vi "CRYSet Sequence Generator Front Panel.vi"(11 "Vi Ref In":refnum<vi> caption="Vi Ref") -> (3 "Vi Ref Out":refnum<vi> caption="Vi Ref")   [LabVIEW 2013]
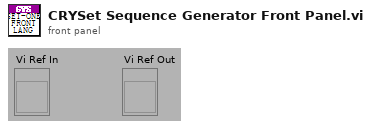
[diagram p1: front panel]
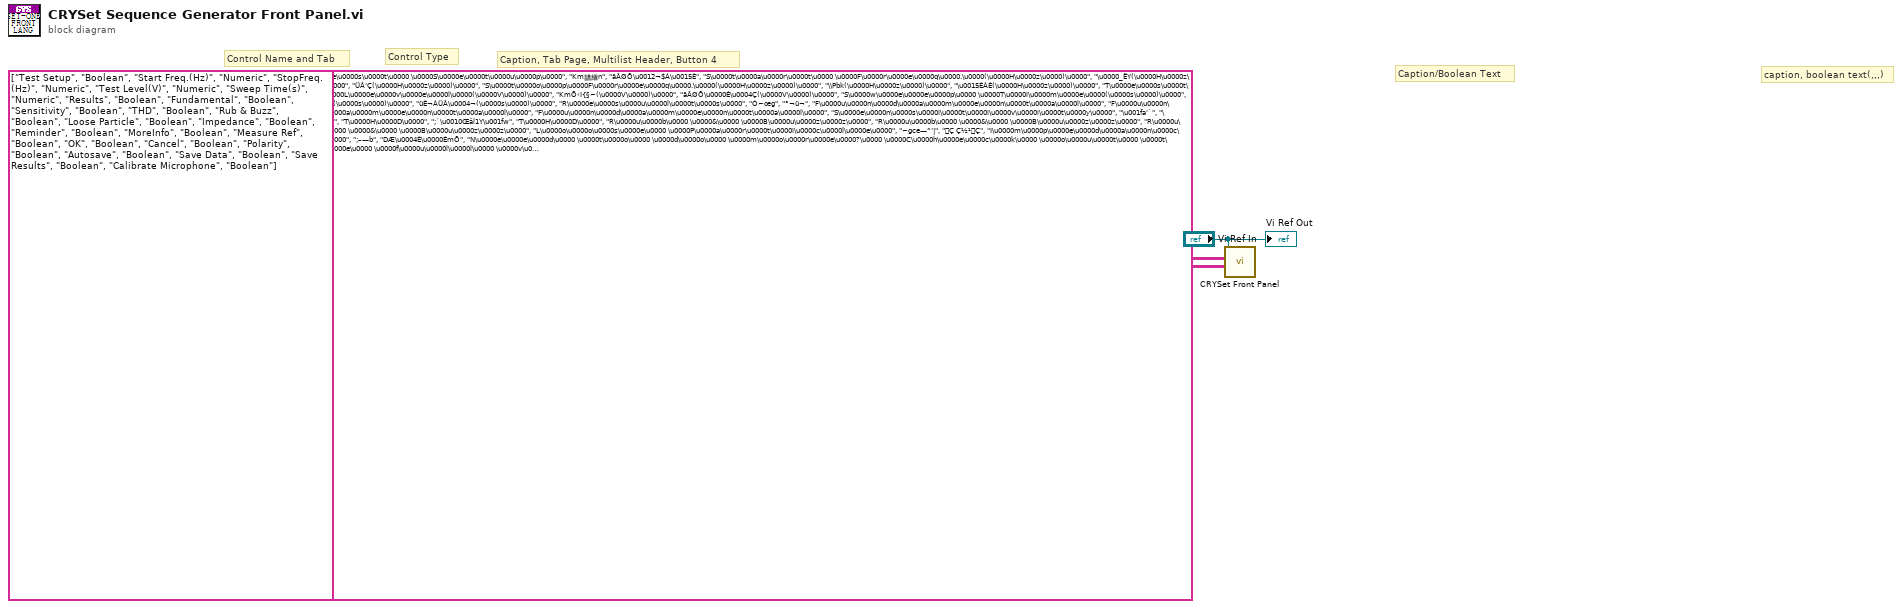
[diagram p0: block diagram]
diagram:
  # "Caption, Tab Page, Multilist Header, Button 4"
  # "Control Type"
  # "Control Name and Tab"
  # "caption, boolean text(,,,)"
  # "Caption/Boolean Text"
  n1 = call "CRYSet Front Panel.vi"("Caption(Boolean Text)"=string[][] [["T\u0000e\u0000s\u0000t\u0000 \u0000S\u0000e\u0000t\u0000u\u0000p\u0000", "Km諎緥n", "äÂØÕ\u0012¬$Á\u0015È"], ["S\u0000t\u0000a\u0000r\u0000t\u0000 \u0000F\u0000r\u0000e\u0000q\u0000.\u0000(\u0000H\u0000z\u0000)\u0000", "\u0000_ËY(\u0000H\u0000z\u0000)\u0000", "ÜÂ‘Ç(\u0000H\u0000z\u0000)\u0000"], ["S\u0000t\u0000o\u0000p\u0000F\u0000r\u0000e\u0000q\u0000.\u0000(\u0000H\u0000z\u0000)\u0000", "\\Pbk(\u0000H\u0000z\u0000)\u0000", "\u0015ÈÀÉ(\u0000H\u0000z\u0000)\u0000"], ["T\u0000e\u0000s\u0000t\u0000 \u0000L\u0000e\u0000v\u0000e\u0000l\u0000(\u0000V\u0000)\u0000", "KmÕ‹I{§~(\u0000V\u0000)\u0000", "äÂØÕ\u0000É\u0004Ç(\u0000V\u0000)\u0000"], ["S\u0000w\u0000e\u0000e\u0000p\u0000 \u0000T\u0000i\u0000m\u0000e\u0000(\u0000s\u0000)\u0000", "kbÏcöeô•(\u0000s\u0000)\u0000", "üÈ¬ÀÜÂ\u0004¬(\u0000s\u0000)\u0000"], ["R\u0000e\u0000s\u0000u\u0000l\u0000t\u0000s\u0000", "Ó~œg", "°¬ü¬"], ["F\u0000u\u0000n\u0000d\u0000a\u0000m\u0000e\u0000n\u0000t\u0000a\u0000l\u0000", "F\u0000u\u0000n\u0000d\u0000a\u0000m\u0000e\u0000n\u0000t\u0000a\u0000l\u0000", "F\u0000u\u0000n\u0000d\u0000a\u0000m\u0000e\u0000n\u0000t\u0000a\u0000l\u0000"], ["S\u0000e\u0000n\u0000s\u0000i\u0000t\u0000i\u0000v\u0000i\u0000t\u0000y\u0000", "\u001fa'`", "\u0010¬Ä³"], ["T\u0000H\u0000D\u0000", ";`\u0010Œâl1Y\u001fw", "T\u0000H\u0000D\u0000"], ["R\u0000u\u0000b\u0000 \u0000&\u0000 \u0000B\u0000u\u0000z\u0000z\u0000", "R\u0000u\u0000b\u0000 \u0000&\u0000 \u0000B\u0000u\u0000z\u0000z\u0000", "R\u0000u\u0000b\u0000 \u0000&\u0000 \u0000B\u0000u\u0000z\u0000z\u0000"], ["L\u0000o\u0000o\u0000s\u0000e\u0000 \u0000P\u0000a\u0000r\u0000t\u0000i\u0000c\u0000l\u0000e\u0000", "~gce—˜’|", "Ç Ç½¹Ç"], ["I\u0000m\u0000p\u0000e\u0000d\u0000a\u0000n\u0000c\u0000e\u0000", ";–—b", "DÆ\u0004È\u0000ÈmÕ"], ["N\u0000e\u0000e\u0000d\u0000 \u0000t\u0000o\u0000 \u0000d\u0000o\u0000 \u0000m\u0000o\u0000r\u0000e\u0000?\u0000 \u0000C\u0000h\u0000e\u0000c\u0000k\u0000 \u0000o\u0000u\u0000t\u0000 \u0000t\u0000h\u0000e\u0000 \u0000f\u0000u\u0000l\u0000l\u0000 \u0000v\u0000e\u0000r\u0000s\u0000i\u0000o\u0000n\u0000\n\u0000o\u0000f\u0000 \u0000C\u0000R\u0000Y\u00006\u00001\u00008\u00001\u0000.\u0000", "\u0000ZPvôf\u001aY\u0017T\u001fÿ\u0000?bv[teHr \u0000\n\u0000vC\u0000R\u0000Y\u00006\u00001\u00008\u00001\u0000\u00020\u0000\u0000", "C\u0000R\u0000Y\u00006\u00001\u00008\u00001\u0000DÆ\u0004È\u0010Óø¼DÇ \u0000¬¹©ÆXÕìÅ \u0000€¬¬ÀXÕÜÂ$¸tº \u0000"], ["C\u0000l\u0000i\u0000c\u0000k\u0000 \u0000f\u0000o\u0000r\u0000 \u0000m\u0000o\u0000r\u0000e\u0000 \u0000i\u0000n\u0000f\u0000o\u0000.\u0000", "¹pûQåg\u000bwæ‹Æ~áOo`", "ìÅ0®|¹ \u0000\u0004²t¹íÂÜÂ$Æ"], ["M\u0000e\u0000a\u0000s\u0000u\u0000r\u0000e\u0000 \u0000R\u0000e\u0000f\u0000e\u0000r\u0000e\u0000n\u0000c\u0000e\u0000 \u0000S\u0000t\u0000a\u0000n\u0000d\u0000a\u0000r\u0000d\u0000", "KmÏ‘ÂS\u0003€\u0007hÆQ", "!Î\u0015È8Ìà¬\\Ô\u0000É"], ["O\u0000K\u0000", "nxš[", "UÖxÇ"], ["C\u0000a\u0000n\u0000c\u0000e\u0000l\u0000", "ÖSˆm", "èÍŒÁ"], ["P\u0000o\u0000l\u0000a\u0000r\u0000i\u0000t\u0000y\u0000", "g'`", "ù­1Á"], ["A\u0000u\u0000t\u0000o\u0000s\u0000a\u0000v\u0000e\u0000", "ê¨RÝOX[", "ÇÙ³ô¼\u0000­"], ["S\u0000a\u0000v\u0000e\u0000 \u0000D\u0000a\u0000t\u0000a\u0000", "ÝOX[penc", "ÇÌ¸ô¼\u0000­"], ["S\u0000a\u0000v\u0000e\u0000 \u0000R\u0000e\u0000s\u0000u\u0000l\u0000t\u0000s\u0000", "ÝOX[Ó~œg", "°¬ü¬ô¼\u0000­"], ["C\u0000a\u0000l\u0000i\u0000b\u0000r\u0000a\u0000t\u0000e\u0000 \u0000M\u0000i\u0000c\u0000r\u0000o\u0000p\u0000h\u0000o\u0000n\u0000e\u0000", "!hÆQ¦žKQÎ˜", "È¹tÇlÐP­\u0000É"]], "Control ID and Type(Label Name, Type)"=string[][] [["Test Setup", "Boolean"], ["Start Freq.(Hz)", "Numeric"], ["StopFreq.(Hz)", "Numeric"], ["Test Level(V)", "Numeric"], ["Sweep Time(s)", "Numeric"], ["Results", "Boolean"], ["Fundamental", "Boolean"], ["Sensitivity", "Boolean"], ["THD", "Boolean"], ["Rub & Buzz", "Boolean"], ["Loose Particle", "Boolean"], ["Impedance", "Boolean"], ["Reminder", "Boolean"], ["MoreInfo", "Boolean"], ["Measure Ref", "Boolean"], ["OK", "Boolean"], ["Cancel", "Boolean"], ["Polarity", "Boolean"], ["Autosave", "Boolean"], ["Save Data", "Boolean"], ["Save Results", "Boolean"], ["Calibrate Microphone", "Boolean"]], "Vi Ref"="Vi Ref In") -> ()  [unwired: 9 in]
  "Vi Ref Out" <- "Vi Ref In"
